vi "Create Motor.vi"(0 "reference in":refnum<class "Gasoline Engine Factory.lvclass">, 11 "Error In":errorcluster) -> (4 "reference out":refnum<class "Gasoline Engine Factory.lvclass">, 6 "Gasoline Motor":refnum<class "IMotor.lvclass">, 15 "Error Out":errorcluster)   [LabVIEW 2024, in "Gasoline Engine Factory.lvclass"]
uses:
  Gasoline Engine Factory.lvclass
  Gasoline Engine Factory.lvclass/Gasoline Engine Factory.ctl
  Product Folder/Gasoline Motor/Gasoline Motor.lvclass
  C:/Users/burakkorkmaz/Desktop/Leveling/labview-desing-patterns/Abstract Factory Pattern/Product Folder/Gasoline Motor/Gasoline Motor.lvclass
  C:/Users/burakkorkmaz/Desktop/Leveling/labview-desing-patterns/Abstract Factory Pattern/Product Folder/IMotor/IMotor.lvclass
  Product Folder/IMotor/IMotor.lvclass
panel:
  # "Connector Pane"
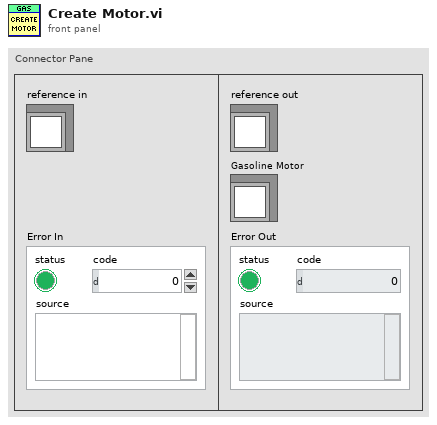
[diagram p1: front panel]
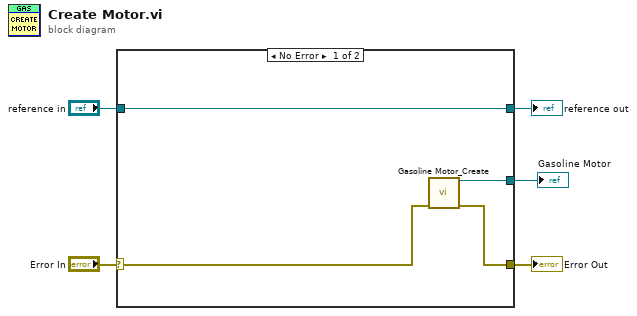
[diagram p0: block diagram]
diagram:
  n1 = case shown="No Error" "Error In" {
    selector: "Error In" -> [w8 w11]
    tunnel: [w7 w11] -> w4
    tunnel: [w9 w10] -> w2
    tunnel: "reference in" -> [w9 w10]
    tunnel: [w6 _] -> w1
    frame No Error {
      n2 = call "Gasoline Motor_Create.vi"("Error In"=w8) -> ("reference out"=w6:refnum<class "Gasoline Motor.lvclass">, "Error Out"=w7:errorcluster)  [unwired: 13 in]
    }
    frame Error {
    }
  }
  "Error Out" <- w4
  "reference out" <- w2
  "Gasoline Motor" <- w1
